vi "Move to point - polar.vi"(11 "Point":T1) -> ()   [LabVIEW 2011]
uses:
  point.ctl
  <vilib>/addons/control/pid/pid.llb/PID (DBL).vi
  <vilib>/Analysis/coordinate.llb/2D Cartesian Coordinate Rotation (Scalar).vi
  <vilib>/Analysis/NI_AALPro.lvlib
  <vilib>/addons/control/pid/NI_PID_pid.lvlib
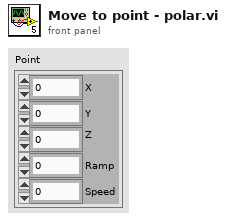
[diagram p1: front panel]
types:
  T1 = typedef "point.ctl" = cluster{"X":dbl, "Y":dbl, "Z":dbl, "Ramp":dbl, "Speed":dbl}
  T2 = typedef "WPI_EncoderDevRef.ctl" = cluster{"DevStatus":errorcluster, "EncoderIndex":T3, "CounterIndex":T4, "DistancePerCount":dbl, "Decoding Type":T5}
  T3 = typedef "FPGA_EncoderIdx.ctl" = enum8{"Enc 0", "Enc 1", "Enc 2", "Enc 3", "Invalid"}
  T4 = typedef "FPGA_CounterCtrSystemIndex.ctl" = enum8{"Ctr 0", "Ctr 1", "Ctr 2", "Ctr 3", "Ctr 4", "Ctr 5", "Ctr 6", "Ctr 7", "Invalid"}
  T5 = typedef "WPI_EncoderType.ctl" = enum16{"1x", "2x", "4x"}
  T6 = typedef "WPI_MotorControlDeviceRef.ctl" = cluster{"DeviceStatus":errorcluster, "Type":enum16{"PWM", "CAN"}, "PWM":cluster{"Digital Module":T7, "PWM Channel":T8, "DeadBand":T9}, "CAN":cluster{"Device Number":u8, "Control Mode":T10, "Semaphore":T11, "Max Vout":dbl}, "Invert":bool, "TransformRef":T12, "InvTransformRef":T12}
  T7 = typedef "FPGA_TypedefDigitalModule.ctl" = enum16{"Digital Module 1", "Digital Module 2"}
  T8 = typedef "FPGA_DIOPWMChannel.ctl" = enum8{"PWM 1", "PWM 2", "PWM 3", "PWM 4", "PWM 5", "PWM 6", "PWM 7", "PWM 8", "PWM 9", "PWM 10", "Invalid"}
  T9 = typedef "WPI_PWMDeadband.ctl" = cluster{"Name":string, "maxPositivePwm":i32, "minPositivePwm":i32, "centerPwm":i32, "maxNegativePwm":i32, "minNegativePwm":i32, "angularRange":u16}
  T10 = typedef "WPI_CANJaguar_ControlMode.ctl" = enum8{"Percent VBus", "Current", "Speed", "Position", "Voltage"}
  T11 = typedef "Semaphore RefNum" = refnum<k1>
  T12 = typedef "WPI_PWMTransform_ConPane.ctl" = refnum<vi>
  T13 = cluster{"proportional gain (Kc)":dbl, "integral time (Ti, min)":dbl, "derivative time (Td, min)":dbl}
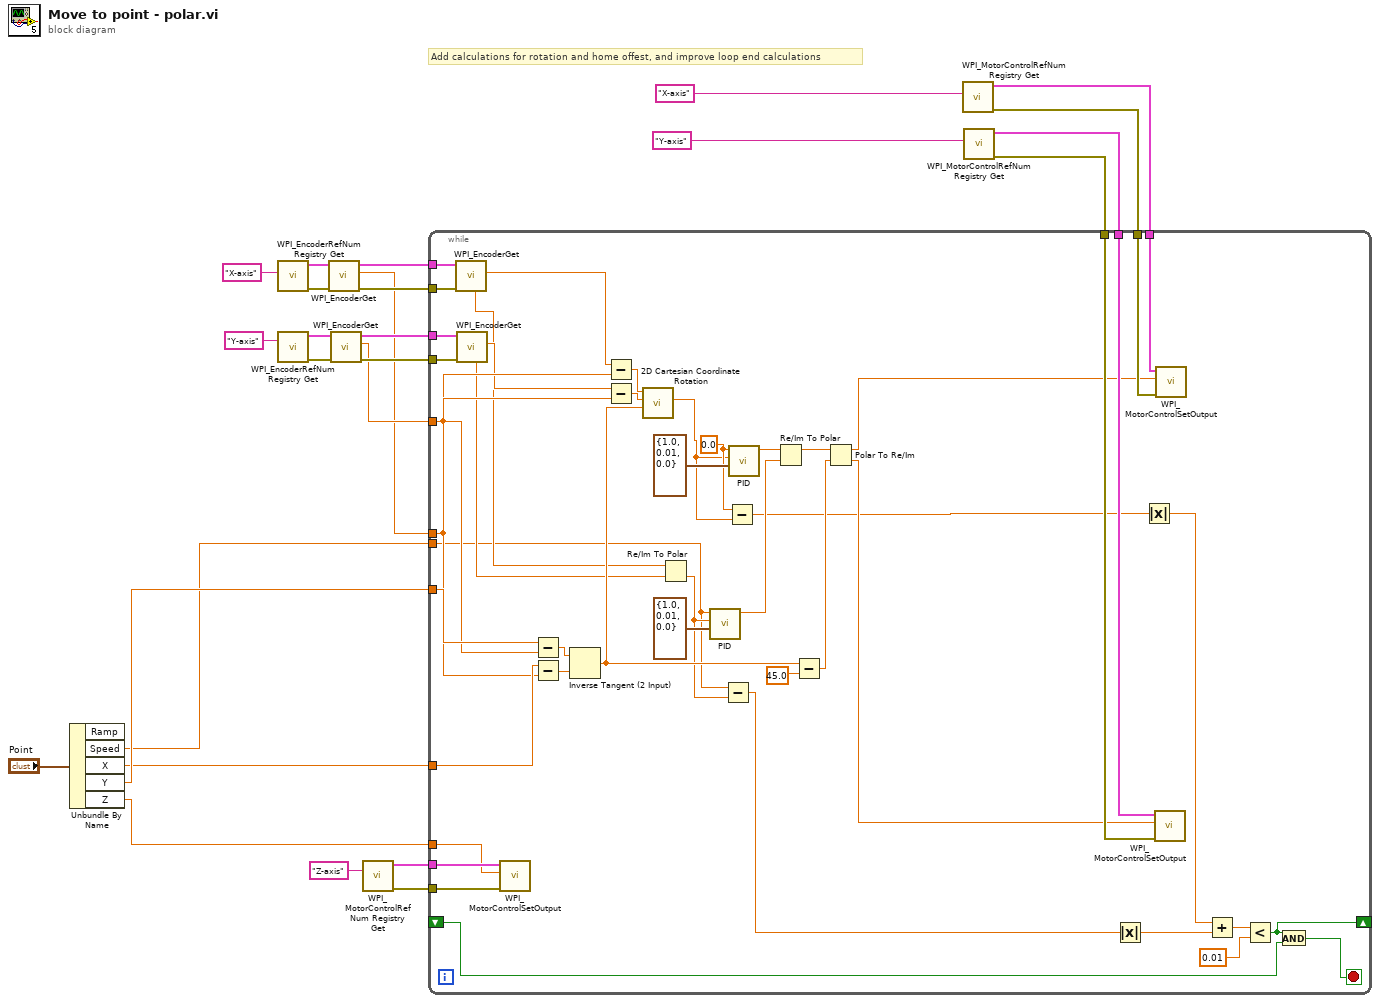
[diagram p0: block diagram]
diagram:
  # "Add calculations for rotation and home offest, and improve loop end calculations"
  n1 = Unbundle By Name("Point") -> ("Speed"=w1:dbl, "X"=w4:dbl, "Y"=w5:dbl, "Z"=w14:dbl)  [unwired: 1 out]
  n2 = call <vilib>:"WPI_EncoderRefNum Registry Get.vi"("refnum name"="X-axis") -> ("error out"=w13:errorcluster, "EncoderDevRef"=w12:T2)  [unwired: 9 in]
  n3 = call <vilib>:"WPI_EncoderRefNum Registry Get.vi"("refnum name"="Y-axis") -> ("error out"=w10:errorcluster, "EncoderDevRef"=w11:T2)  [unwired: 9 in]
  n4 = call <vilib>:"WPI_EncoderGet.vi"("error in (no error)"=w13, "EncoderDevRef"=w12) -> ("error out"=w7:errorcluster, "Distance"=w2:dbl, "EncoderDevRef"=w6:T2)  [unwired: 4 in, 3 out]
  n5 = call <vilib>:"WPI_EncoderGet.vi"("error in (no error)"=w10, "EncoderDevRef"=w11) -> ("error out"=w8:errorcluster, "Distance"=w3:dbl, "EncoderDevRef"=w9:T2)  [unwired: 4 in, 3 out]
  n6 = call <vilib>:"WPI_MotorControlRefNum Registry Get.vi"("refnum name"="Z-axis") -> ("error out"=w16:errorcluster, "MotorControlDevRef"=w17:T6)  [unwired: 9 in]
  n7 = call <vilib>:"WPI_MotorControlRefNum Registry Get.vi"("refnum name"="X-axis") -> ("error out"=w21:errorcluster, "MotorControlDevRef"=w22:T6)  [unwired: 9 in]
  n8 = call <vilib>:"WPI_MotorControlRefNum Registry Get.vi"("refnum name"="Y-axis") -> ("error out"=w18:errorcluster, "MotorControlDevRef"=w19:T6)  [unwired: 9 in]
  n9 = while {
    tunnel: w7 -> [w72]
    tunnel: w6 -> [w71]
    tunnel: w9 -> [w70]
    tunnel: w8 -> [w69]
    shift-right: [w66] -> _
    shift-left: _ -> [w65]
    tunnel: w22 -> [w64]
    tunnel: w21 -> [w55]
    tunnel: w19 -> [w63]
    tunnel: w18 -> [w62]
    tunnel: w17 -> [w61]
    tunnel: w16 -> [w60]
    tunnel: w14 -> [w59]
    tunnel: w5 -> [w42]
    tunnel: w4 -> [w41]
    tunnel: w3 -> [w38]
    tunnel: w2 -> [w37]
    tunnel: w1 -> [w27]
    stop <- w56 stop-if-true
    w32 = 0.0 ("setpoint")
    n10 = call <vilib>:"WPI_EncoderGet.vi"("error in (no error)"=w72, "EncoderDevRef"=w71) -> ("Distance"=w36:dbl, "Rate"=w34:dbl)  [unwired: 4 in, 4 out]
    n11 = call <vilib>:"WPI_EncoderGet.vi"("error in (no error)"=w69, "EncoderDevRef"=w70) -> ("Distance"=w35:dbl, "Rate"=w33:dbl)  [unwired: 4 in, 4 out]
    n12 = call <vilib>:"WPI_MotorControlSetOutput.vi"("error in (no error)"=w60, "Output"=w59, "MotorControlDevRef"=w61) -> ()  [unwired: 7 in, 2 out]
    n13 = Subtract(x=w42, y=w38) -> (x-y=w53:dbl)
    n14 = Subtract(x=w41, y=w37) -> (x-y=w54:dbl)
    n15 = Inverse Tangent (2 Input)(1:w54, 2:w53) -> (0:w48:dbl)
    n16 = Subtract(x=w36, y=w37) -> (x-y=w52:dbl)
    n17 = Subtract(x=w35, y=w38) -> (x-y=w51:dbl)
    n18 = call-poly <vilib>:"2D Cartesian Coordinate Rotation.vi"("theta"=w48, "y"=w51, "x"=w52) -> ("y out"=w31:dbl)  [unwired: 6 in, 2 out]
    n19 = Re/Im To Polar(2:w33, 3:w34) -> (0:w30:dbl)  [unwired: 1 out]
    n20 = call-poly <vilib>:"PID.vi"("PID gains"=T13 {"proportional gain (Kc)"=1.0, "integral time (Ti, min)"=0.01, "derivative time (Td, min)"=0.0}, "process variable"=w30, "setpoint"=w27) -> ("output"=w43:dbl)  [unwired: 7 in, 1 out]
    n21 = Subtract(x=w27, y=w30) -> (x-y=w29:dbl)
    n22 = Subtract(x=w32, y=w31) -> (x-y=w28:dbl)
    n23 = call-poly <vilib>:"PID.vi"("PID gains"=T13 {"proportional gain (Kc)"=1.0, "integral time (Ti, min)"=0.01, "derivative time (Td, min)"=0.0}, "process variable"=w31, "setpoint"=w32) -> ("output"=w45:dbl)  [unwired: 7 in, 1 out]
    n24 = Re/Im To Polar(2:w43, 3:w45) -> (1:w47:dbl)  [unwired: 1 out]
    n25 = Subtract(x=w48, y=45.0) -> (x-y=w49:dbl)
    n26 = Polar To Re/Im(2:w49, 3:w47) -> (0:w39:dbl, 1:w40:dbl)
    n27 = Absolute Value(x=w29) -> (abs(x)=w58:dbl)
    n28 = Absolute Value(x=w28) -> (abs(x)=w57:dbl)
    n29 = call <vilib>:"WPI_MotorControlSetOutput.vi"("error in (no error)"=w62, "Output"=w39, "MotorControlDevRef"=w63) -> ()  [unwired: 7 in, 2 out]
    n30 = call <vilib>:"WPI_MotorControlSetOutput.vi"("error in (no error)"=w55, "Output"=w40, "MotorControlDevRef"=w64) -> ()  [unwired: 7 in, 2 out]
    n31 = Add(x=w57, y=w58) -> (x+y=w68:dbl)
    n32 = Less?(x=w68, y=0.01) -> (x < y?=w66:bool)
    n33 = And(x=w66, y=w65) -> (x .and. y?=w56:bool)
  }
